vi "BluetoothSettings.vi"(11 "notifier":refnum<notifier>) -> ()   [LabVIEW 2013, in "main.lvlib"]
uses:
  main.lvlib
  Controls/Enum Variables.ctl
  Controls/Enum Save Action Events.ctl
  <vilib>/GPower/String/GPString.lvlib
panel:
  in  "EditBluetoothSettingsBtn":bool
  in  "CheckLicenseBtn":bool
  out "BTDeviceTable":string[][](table) caption="Registrerede apparater"
  in  "BTLicenseStr":string caption="Licens"
  out "BT SerialLabel":string="Bluetooth Licens" caption="generalSettingsString"
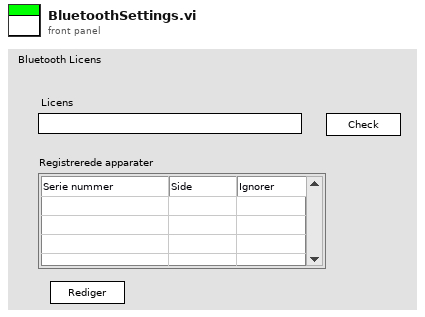
[diagram p1: front panel]
types:
  T1 = typedef "main.lvlib/Enum Variables.ctl" = enum16{"SetAcqFilter", "GetAcqFilter", "Set Filter", "Get Filter", "Set Height", "Get Height", "Set Recorded Height", "Get Recorded Height", "Set Blue Pressure", "Get Blue Pressure", "Set Red Pressure", "Get Red Pressure", "Init", "Reset Pressure", "Set Red Cursors", "Get Red Cursors", "Set Blue Cursors", "Get Blue Cursors", "Set Language", "Get Language", "Set Active Graphs", "Get ActiveGraphs", "Set Method", "Get Method", "Set Encryption", "Get Encryption", "Set ExcelVersion", "Get ExcelVersion", "Set DICOM Avail", "Get DICOM Avail", "Set DICOM Encode", "Get DICOM Encode", "Set JournalExport", "Get JournalExport", "Set Sequence", "Get Sequence", "Set DAQ Connected", "Get DAQ Connected", "Set Current Graph", "Get Current Graph", "Set General Settings", "Get Hyphenation", "Set Arm Calc Method", "Get Arm Calc Method", "Set Dicom Tags", "Get Dicom Tags", "Set BT Serial", "Get BT Serial", "Set BT Accepted Serials", "Get BT Accepted Serials", "Get BT License", "Set BT License"}
  T2 = typedef "main.lvlib/Enum Save Action Events.ctl" = enum16{"LoadReportPath", "SaveReportPath", "Load Graph Path", "Save Graph Path", "LoadDataPath", "SaveDataPath", "Load Template Path", "Save Template Path", "Load PressureFactor", "Save PressureFactor", "Init", "Load Listbox", "Save Listbox", "LoadHospInfo", "SaveHospInfo", "Load DICOM Activation", "Save DICOM Activation", "LoadDICOMInfoWL", "SaveDICOMInfoWL", "LoadDICOMInfoPACS", "SaveDICOMInfoPACS", "Load ArmCalcMethod", "Save ArmCalcMethod", "LoadItemTags", "SaveItemTags", "LoadDICOMEncoding", "SaveDICOMEncoding", "LoadJournalType", "SaveJournalType", "LoadAcqFilterType", "SaveAcqFilterType", "Load Sequence", "Save Sequence", "Load Acquisition Mode", "Save Acquisition Mode", "Load General Settings", "Save General Settings", "Load Language", "Save Language", "Load Dicom Tags", "Save Dicom Tags", "Load BT Serial", "Save BT Serial", "Load BT License", "Save BT License"}
  T3 = cluster{"Serial":string, "Side":string, "Ignorer?":bool}
  T4 = cluster{"Serial":string, "Side":string, "Ignorer?":bool}[]
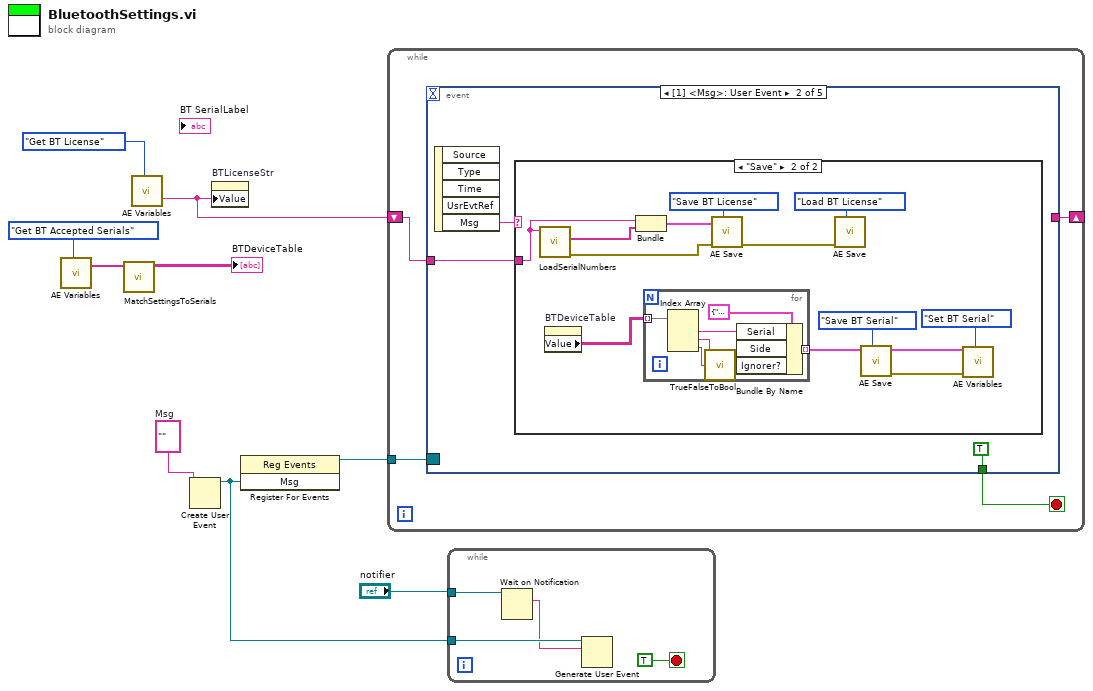
[diagram p0: block diagram]
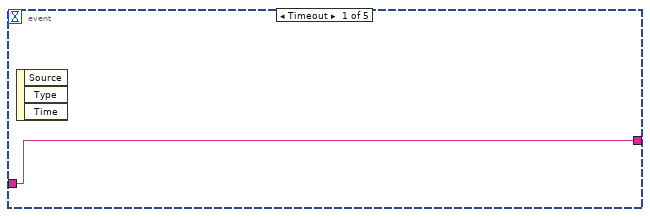
[diagram p2: hidden frame]
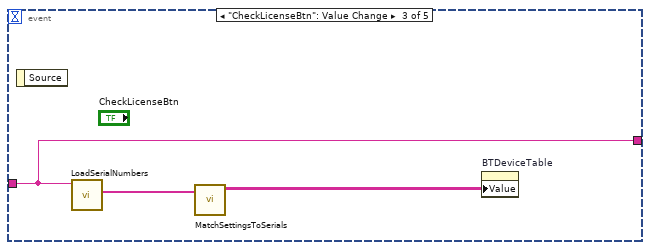
[diagram p4: hidden frame]
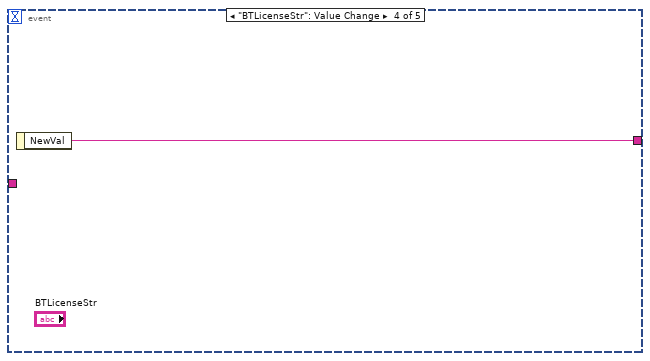
[diagram p5: hidden frame]
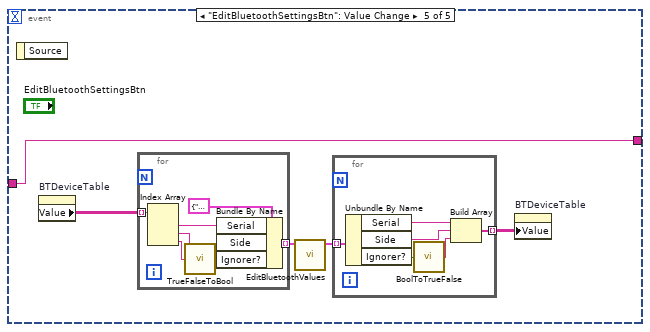
[diagram p6: hidden frame]
diagram:
  w8 = ""  # Msg
  n1 = call "AE Variables.vi"("Action"=Enum_Variables."Get BT Accepted Serials") -> ("stringArray"=w2:string[])  [unwired: 11 in, 7 out]
  n2 = call "MatchSettingsToSerials.vi"("Serials"=w2) -> ("Array"=→"BTDeviceTable":string[][])  [unwired: 10 in]
  n3 = call "AE Variables.vi"("Action"=Enum_Variables."Get BT License") -> ("String"=w4:string)  [unwired: 11 in, 7 out]
  n4 = Create User Event(user event datatype=w8) -> (user event=w7:refnum<user-event>)  [unwired: 1 in, 1 out]
  n5 = property on="BTLicenseStr" class="Str"("Value"=w4) -> ()  [unwired: 2 in, 2 out]
  n6 = register-events(w7) -> (reference out=w5:refnum<event-registration>)  [unwired: 2 in, 1 out]
  n7 = while {
    tunnel: w5 -> [w13]
    shift-right: [w10] -> _
    shift-left: w4 -> [w11]
    stop <- w12 stop-if-true
    n8 = event shown="[1] <Msg>: User Event" {
      selector: w13 -> [_ _ _ _ _]
      dyn-events: _ -> [_ _ _ _ _]
      timeout: _ -> [_ _ _ _ _]
      tunnel: [_ TRUE _ _ _] -> w12
      tunnel: w11 -> [w14 w15 w39 _ w43]
      tunnel: [w14 _ w39 w40 w43] -> w10
      event Timeout {
        n9 = event-data() -> ()  [unwired: 1 in, 3 out]
      }
      event User Event {
        n10 = event-data() -> ("Msg"=w17:string)  [unwired: 1 in, 4 out]
        n11 = case shown="\"Save\"" w17 {
          tunnel: w15 -> [_ w24]
          frame "Cancel", Default {
          }
          frame "Save" {
            n12 = call "LoadSerialNumbers.vi"("License"=w24) -> ("error out"=w26:errorcluster, "Serials"=w25:string[])  [unwired: 8 in, 1 out]
            n13 = property on="BTDeviceTable" class="Tbl (strict)"() -> ("Value"=w22:string[][])  [unwired: 2 in, 2 out]
            n14 = Bundle("String"=w24, "Serials"=w25) -> (w23:cluster{"String":string, "Serials":string[]})  [unwired: 1 in]
            n15 = for {
              tunnel: w22 -> [w35] mode=indexing
              tunnel: [w31] -> w19 mode=indexing
              n16 = Index Array(array=w35) -> (element #1=w34:string, element #2=w33:string, element #3=w32:string)  [unwired: 3 in]
              n17 = call <vilib>:"TrueFalseToBool.vi"("String"=w32) -> ("Boolean"=w36:bool)
              n18 = Bundle By Name(cluster=T3 {"Serial"="", "Side"="", "Ignorer?"=FALSE} ("Cluster"), "Serial"=w34, "Side"=w33, "Ignorer?"=w36) -> (w31:T3)
            }
            n19 = call "AE Save.vi"("error in (no error)"=w26, "Variant In"=w23, "Action"=Enum_Save_Action_Events."Save BT License") -> ("error out"=w27:errorcluster)  [unwired: 6 in, 1 out]
            n20 = call "AE Save.vi"("error in (no error)"=w27, "Action"=Enum_Save_Action_Events."Load BT License") -> ()  [unwired: 7 in, 2 out]
            n21 = call "AE Save.vi"("Variant In"=w19, "Action"=Enum_Save_Action_Events."Save BT Serial") -> ("error out"=w18:errorcluster)  [unwired: 7 in, 1 out]
            n22 = call "AE Variables.vi"("VariantIn"=w19, "error in (no error)"=w18, "Action"=Enum_Variables."Set BT Serial") -> ()  [unwired: 9 in, 8 out]
          }
        }
      }
      event "CheckLicenseBtn": Value Change {
        n23 = event-data() -> ()  [unwired: 1 in, 1 out]
        n24 = call "LoadSerialNumbers.vi"("License"=w39) -> ("Serials"=w38:string[])  [unwired: 8 in, 2 out]
        n25 = call "MatchSettingsToSerials.vi"("Serials"=w38) -> ("Array"=w37:string[][])  [unwired: 10 in]
        n26 = property on="BTDeviceTable" class="Tbl (strict)"("Value"=w37) -> ()  [unwired: 2 in, 2 out]
      }
      event "BTLicenseStr": Value Change {
        n27 = event-data() -> ("NewVal"=w40:string)  [unwired: 1 in]
      }
      event "EditBluetoothSettingsBtn": Value Change {
        n28 = event-data() -> ()  [unwired: 1 in, 1 out]
        n29 = property on="BTDeviceTable" class="Tbl (strict)"() -> ("Value"=w45:string[][])  [unwired: 2 in, 2 out]
        n30 = for {
          tunnel: w45 -> [w57] mode=indexing
          tunnel: [w53] -> w44 mode=indexing
          n31 = Index Array(array=w57) -> (element #1=w56:string, element #2=w55:string, element #3=w54:string)  [unwired: 3 in]
          n32 = call <vilib>:"TrueFalseToBool.vi"("String"=w54) -> ("Boolean"=w58:bool)
          n33 = Bundle By Name(cluster=T3 {"Serial"="", "Side"="", "Ignorer?"=FALSE} ("Cluster"), "Serial"=w56, "Side"=w55, "Ignorer?"=w58) -> (w53:T3)
        }
        n34 = call "EditBluetoothValues.vi"("In array"=w44) -> ("Out array"=w42:T4)  [unwired: 10 in]
        n35 = for {
          tunnel: w42 -> [w51] mode=indexing
          tunnel: [w46] -> w41 mode=indexing
          n36 = Unbundle By Name(w51) -> ("Serial"=w47:string, "Side"=w48:string, "Ignorer?"=w50:bool)
          n37 = call <vilib>:"BoolToTrueFalse.vi"("Boolean"=w50) -> ("String"=w49:string)
          n38 = Build Array(w47, w48, w49) -> (w46:string[])
        }
        n39 = property on="BTDeviceTable" class="Tbl (strict)"("Value"=w41) -> ()  [unwired: 2 in, 2 out]
      }
    }
  }
  n40 = while {
    tunnel: "notifier" -> [w62]
    tunnel: w7 -> [w60]
    stop <- TRUE stop-if-true
    n41 = Wait on Notification(notifier=w62) -> (notification=w59:string)  [unwired: 3 in, 3 out]
    n42 = Generate User Event(user event=w60, event data cluster=w59) -> ()  [unwired: 2 in, 2 out]
  }
